vi "NI PXI-4072 DMM Initialization VI.vi"(8 "error in (no error)":errorcluster, 10 "Custom XML":string, 11 "Device Item Ref in":T1 format="%.0x") -> (0 "error out":errorcluster, 3 "Device Item Ref out":T1 format="%.0x")   [LabVIEW 2009, in "NI PXI-4072 DMM Custom Device.lvlib"]
uses:
  NI PXI-4072 DMM Custom Device.lvlib
  <vilib>/NI VeriStand/Custom Device API/Custom Device Item Ref.ctl
  <vilib>/NI VeriStand/Custom Device API/Custom Device Channel.ctl
  <vilib>/NI VeriStand/Custom Device API/Custom Device Channel Type.ctl
  <vilib>/NI VeriStand/Custom Device API/Custom Device Loop Type.ctl
  <vilib>/NI VeriStand/Custom Device API/Custom Device API.lvlib
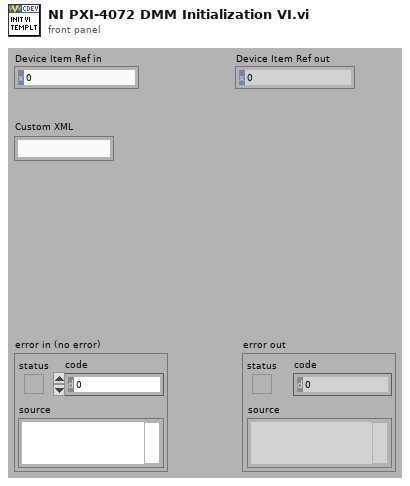
[diagram p1: front panel]
types:
  T1 = typedef "Custom Device API.lvlib/Custom Device Item Ref.ctl" = u64
  T2 = typedef "Custom Device API.lvlib/Custom Device Channel.ctl" = cluster{"Type":T3, "Units":string, "Default Value":dbl, "Faultable":bool, "Scalable":bool}
  T3 = typedef "Custom Device API.lvlib/Custom Device Channel Type.ctl" = enum16{"Input", "Output"}
  T4 = typedef "Custom Device API.lvlib/Custom Device Loop Type.ctl" = enum32{"While Loop", "Timed Loop"}
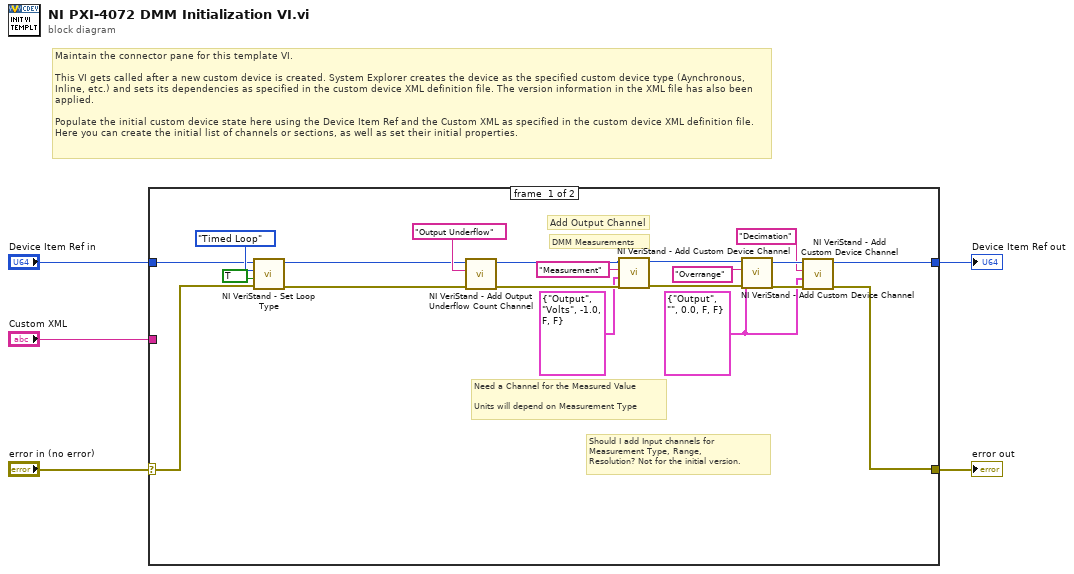
[diagram p0: block diagram]
diagram:
  # "Maintain the connector pane for this template VI.\n\nThis VI gets called after a new custom device is created. System Explorer creates the device as the specified custom device type (Aynchronous, Inline, etc.) and sets its dependencies as specified in the custom device XML definition file. The version information in the XML file has also been applied.\n\nPopulate the initial custom device state here using the Device Item Ref and the Custom XML as specified in the custom device XML definition file. Here you can create the initial list of channels or sections, as well as set their initial properties."
  n1 = case shown="No Error" "error in (no error)" {
    selector: "error in (no error)" -> [w22 w27]
    tunnel: [w8 w27] -> w5
    tunnel: [w9 w26] -> w3
    tunnel: "Device Item Ref in" -> [w23 w26]
    tunnel: "Custom XML" -> [_ _]
    frame #0 {
      w10 = T2 {"Type"=enum."Output", "Units"="", "Default Value"=0.0, "Faultable"=FALSE, "Scalable"=FALSE} ("Channel")
      # "Need a Channel for the Measured Value\n\nUnits will depend on Measurement Type"
      # "Should I add Input channels for\nMeasurement Type, Range,\nResolution? Not for the initial version."
      # "DMM Measurements"
      # "Add Output Channel"
      n2 = call <vilib>:"NI VeriStand - Set Loop Type.vi"("error in (no error)"=w22, "Use Device Clock (Timed Loops only)"=TRUE, "Loop type"=Custom_Device_Loop_Type."Timed Loop", "Device Ref in"=w23) -> ("error out"=w6:errorcluster, "Device Ref out"=w7:T1)  [unwired: 6 in]
      n3 = call <vilib>:"NI VeriStand - Add Output Underflow Count Channel.vi"("error in (no error)"=w6, "Channel Name"="Output Underflow", "Parent Ref in"=w7) -> ("error out"=w19:errorcluster, "Parent Ref out"=w20:T1)  [unwired: 6 in, 1 out]
      n4 = call <vilib>:"NI VeriStand - Add Custom Device Channel.vi"("error in (no error)"=w19, "Channel"=T2 {"Type"=enum."Output", "Units"="Volts", "Default Value"=-1.0, "Faultable"=FALSE, "Scalable"=FALSE}, "Channel Name"="Measurement", "Parent Ref in"=w20) -> ("error out"=w15:errorcluster, "Parent Ref out"=w14:T1)  [unwired: 5 in, 1 out]
      n5 = call <vilib>:"NI VeriStand - Add Custom Device Channel.vi"("error in (no error)"=w15, "Channel"=w10, "Channel Name"="Overrange", "Parent Ref in"=w14) -> ("error out"=w13:errorcluster, "Parent Ref out"=w12:T1)  [unwired: 5 in, 1 out]
      n6 = call <vilib>:"NI VeriStand - Add Custom Device Channel.vi"("error in (no error)"=w13, "Channel"=w10, "Channel Name"="Decimation", "Parent Ref in"=w12) -> ("error out"=w8:errorcluster, "Parent Ref out"=w9:T1)  [unwired: 5 in, 1 out]
    }
    frame #1 {
    }
  }
  "error out" <- w5
  "Device Item Ref out" <- w3
